vi "Pulse Test Configuration.vi"(0 "RFmx session in":refnum<k21>, 5 "Test Configuration":T1, 11 "error in":errorcluster) -> (4 "RFmx session out":refnum<k21>, 15 "error out":errorcluster)   [LabVIEW 2023]
uses:
  Controls/Test Config - Pulse.ctl
  <resource>/objmgr/RFmxPulse.rc
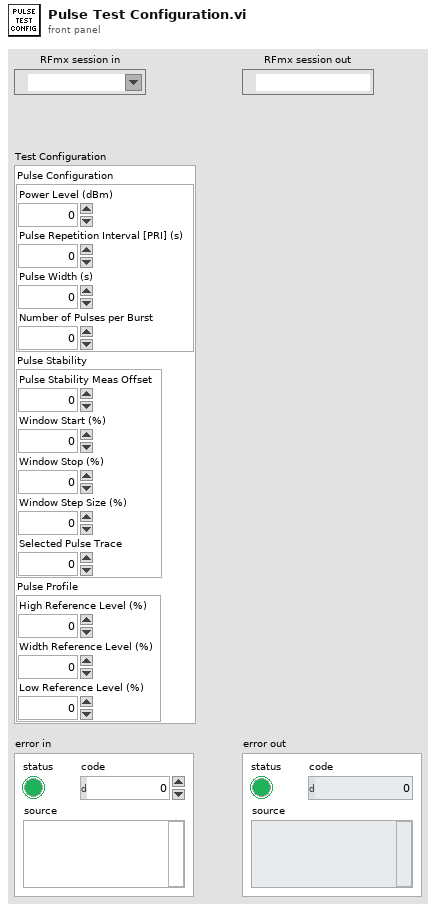
[diagram p1: front panel]
types:
  T1 = typedef "Test Config - Pulse.ctl" = cluster{"Pulse Configuration":cluster{"Power Level (dBm)":dbl, "Pulse Repetition Interval [PRI] (s)":dbl, "Pulse Width (s)":dbl, "Number of Pulses per Burst":u32}, "Pulse Stability":cluster{"Pulse Stability Meas Offset":i32, "Window Start (%)":dbl, "Window Stop (%)":dbl, "Window Step Size (%)":dbl, "Selected Pulse Trace":i32}, "Pulse Profile":cluster{"High Reference Level (%)":dbl, "Width Reference Level (%)":dbl, "Low Reference Level (%)":dbl}}
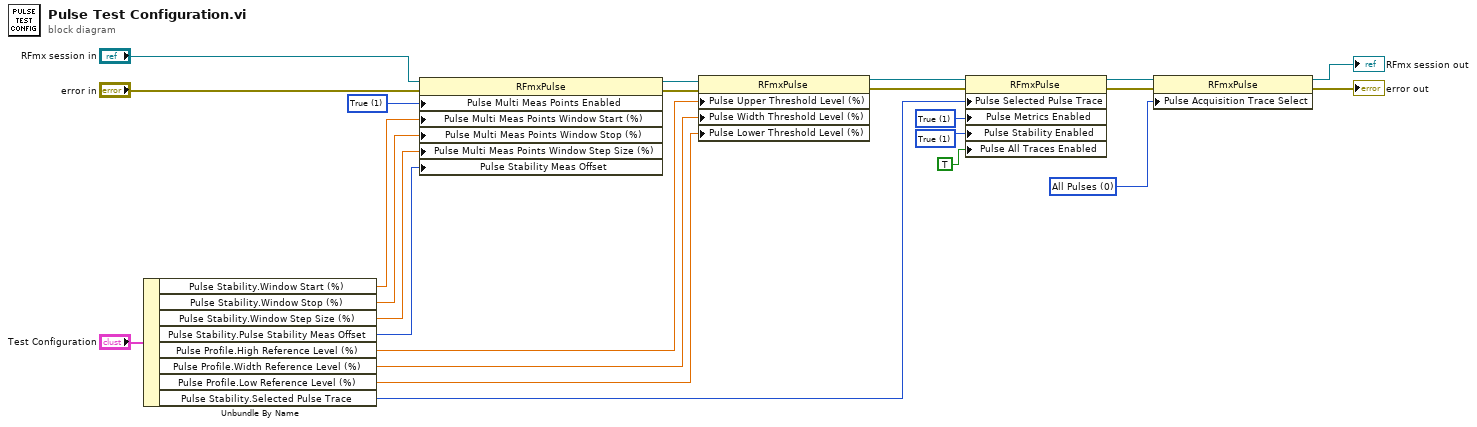
[diagram p0: block diagram]
diagram:
  w1 = 0 items=["All Pulses", "Subset"] ("Pulse Acquisition Trace Select")
  w20 = 1 items=["False", "True"] ("Pulse Multi Meas Points Enabled")
  w23 = 1 items=["False", "True"] ("Pulse Stability Enabled")
  w24 = 1 items=["False", "True"] ("Pulse Metrics Enabled")
  n1 = Unbundle By Name("Test Configuration") -> ("Pulse Stability.Window Start (%)"=w11:dbl, "Pulse Stability.Window Stop (%)"=w12:dbl, "Pulse Stability.Window Step Size (%)"=w13:dbl, "Pulse Stability.Pulse Stability Meas Offset"=w10:i32, "Pulse Profile.High Reference Level (%)"=w9:dbl, "Pulse Profile.Width Reference Level (%)"=w8:dbl, "Pulse Profile.Low Reference Level (%)"=w7:dbl, "Pulse Stability.Selected Pulse Trace"=w6:i32)
  n2 = property class="RFmxPulse"(reference="RFmx session in", error in="error in", "Pulse Multi Meas Points Enabled"=w20, "Pulse Multi Meas Points Window Start (%)"=w11, "Pulse Multi Meas Points Window Stop (%)"=w12, "Pulse Multi Meas Points Window Step Size (%)"=w13, "Pulse Stability Meas Offset"=w10) -> (reference out=w22:refnum<k21>, error out=w21:errorcluster)
  n3 = property class="RFmxPulse"(reference=w22, error in=w21, "Pulse Upper Threshold Level (%)"=w9, "Pulse Width Threshold Level (%)"=w8, "Pulse Lower Threshold Level (%)"=w7) -> (reference out=w19:refnum<k21>, error out=w18:errorcluster)
  n4 = property class="RFmxPulse"(reference=w19, error in=w18, "Pulse Selected Pulse Trace"=w6, "Pulse Metrics Enabled"=w24, "Pulse Stability Enabled"=w23, "Pulse All Traces Enabled"=TRUE) -> (reference out=w4:refnum<k21>, error out=w5:errorcluster)
  n5 = property class="RFmxPulse"(reference=w4, error in=w5, "Pulse Acquisition Trace Select"=w1) -> (reference out=→"RFmx session out":refnum<k21>, error out=→"error out":errorcluster)
